vi "CRYGraph Digital Window.vi"() -> ()   [LabVIEW 2013]
uses:
  Control/CRYFlag Cluster.ctl
  <vilib>/Utility/miscctls.llb/LVRowAndColumnTypeDef.ctl
  <vilib>/Utility/miscctls.llb/LVRectTypeDef.ctl
  SubVI/CRYData View Global.vi
  SubVI/CRYMain Sub Window Global.vi
  CRYCurveLibrary/Global/CRYCurve Library Global.vi
panel:
  out "LegendVScrollShow":bool=TRUE
  in  "LoadFinish":bool
  in  "ScaleFitY":bool
  in  "ScaleFitX":bool
  in  "ToolbarUpdate":bool
  in  "PaletteShow":bool
  out "PropertyTab":string
  in  "OpenProperty":bool
  out "Event Name":string
  out "Test":string
  in  "Cursor":string[][](table)
  out "Cursor Ref":refnum<vi>
  out "Queue Name":string
  in  "StateOut":bool
  in  "CursorShow":bool
  out "Graph Ref":refnum<vi>
  out "Digital Graph":digitalwaveform[](graph)
  in  "LegendShow":bool
  out "Legend Ref":refnum<vi>
  out "Title Name":string
  out "OldRow":i32
  out "TotalPlot":u32
  out "Graph Number":i32
  in  "stop":bool
  in  "ColorBox":u32(colorbox)
  in  "Legend":i32(listbox)
  in  "GraphType":string
types:
  T1 = typedef "CRYFlag Cluster.ctl" = cluster{"LegendShow":bool, "CellClick":bool, "Total Number":bool, "ScaleFitX":bool, "ScaleFitY":bool, "MapModeX":u8, "MapModeY":u8, "CursorShow":bool, "MagnitudeShow":bool, "PreviewShow":bool, "CursorEnabled":bool, "IntensityShow":bool, "PaletteShow":bool, "PhaseShow":bool, "XYShow":bool, "FrequencyShow":bool, "LegendVScrollShow":bool, "FrequencyVScrollShow":bool}
  T2 = cluster{"DisplayTitle":string, "DataViewTitle":string, "DataType":string, "XAxisLabel":string, "YAxisLabel":string, "GraphData":variant}
  T3 = typedef "CRYGraph Event.ctl" = cluster{"EvenName":string, "TitleName":string, "GraphName":string, "GraphType":string, "Data":variant, "Queue Name":string, "DataView Number":i32}
  T4 = enum16{"Curves", "Values", "Results", "WFM", "Others"}
  T5 = typedef "LVRowAndColumnTypeDef.ctl" = cluster{"Row":i32, "Column":i32}
  T6 = typedef "LVRectTypeDef.ctl" = cluster{"Left":i16, "Top":i16, "Right":i16, "Bottom":i16}
  T7 = typedef "LVPoint32TypeDef.ctl" = cluster{"Horizontal":i32, "Vertical":i32}
  T8 = typedef "LVBoundsTypeDef.ctl" = cluster{"Width":u32, "Height":u32}
  T9 = typedef "LVPositionTypeDef.ctl" = cluster{"Left":i32, "Top":i32}
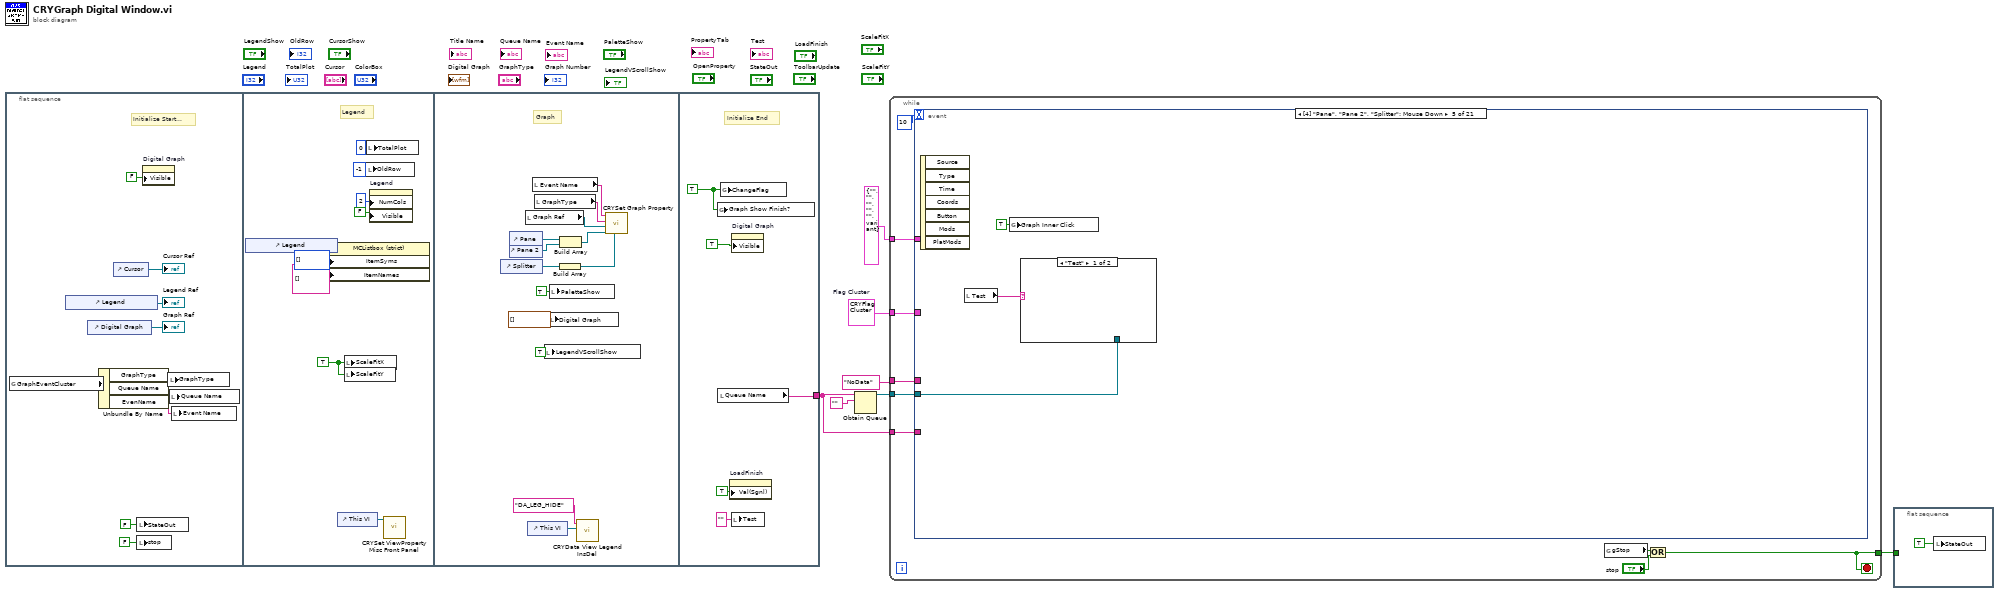
[diagram p0: block diagram]
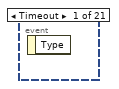
[diagram p2: hidden frame]
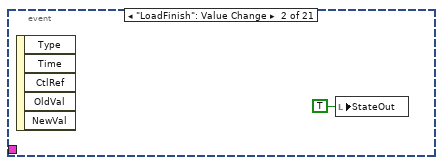
[diagram p3: hidden frame]
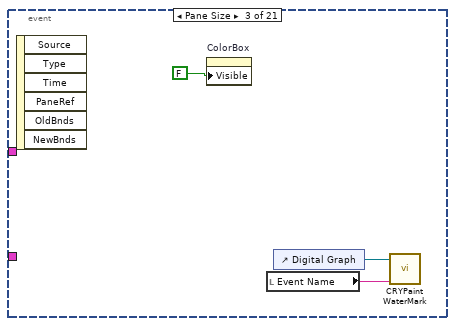
[diagram p4: hidden frame]
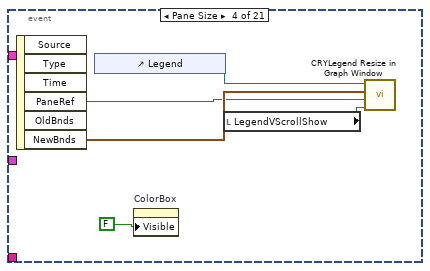
[diagram p5: hidden frame]
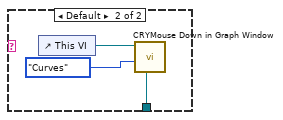
[diagram p6: hidden frame]
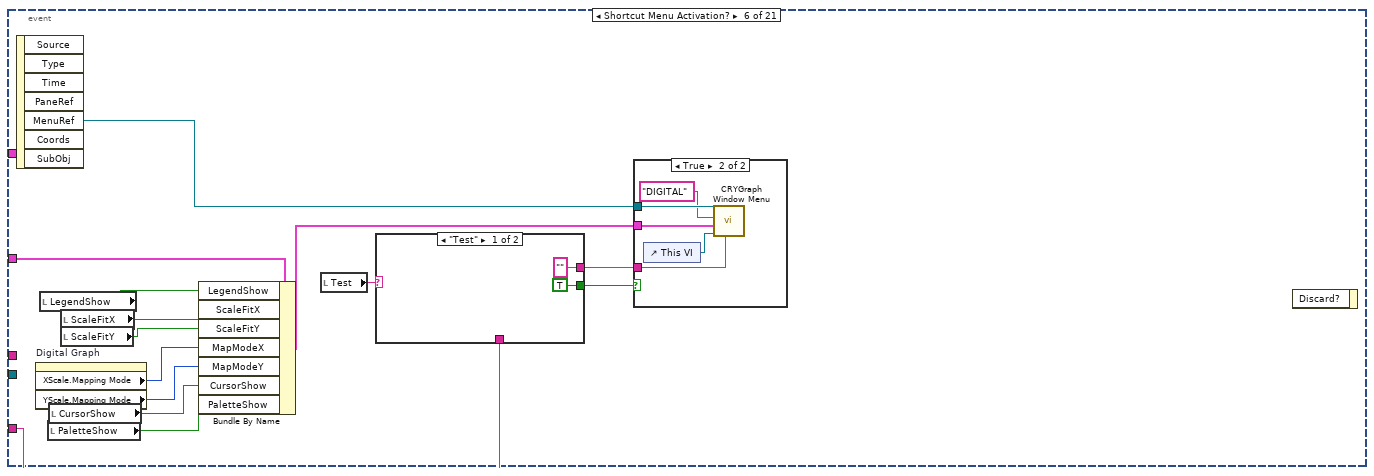
[diagram p7: hidden frame]
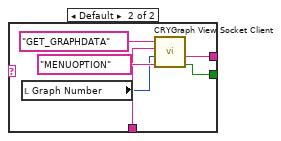
[diagram p8: hidden frame]
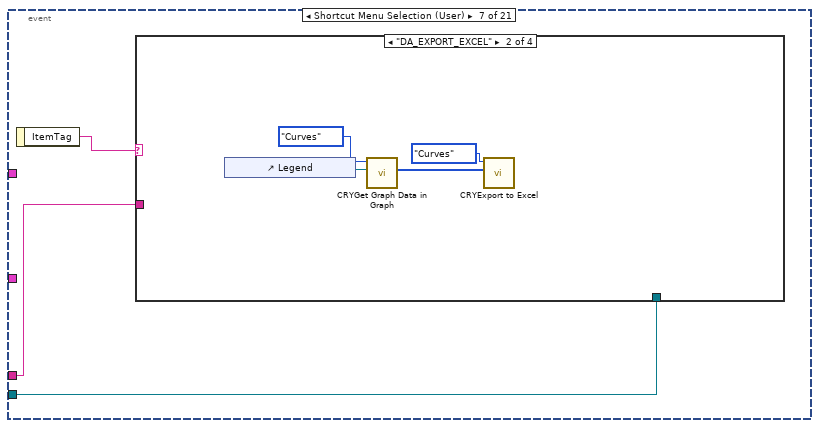
[diagram p10: hidden frame]
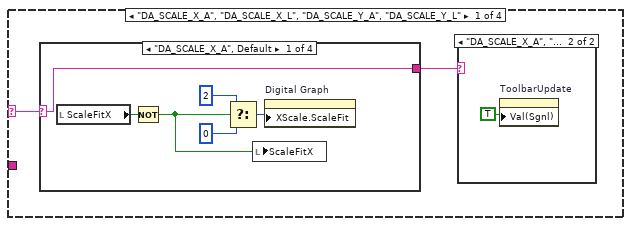
[diagram p11: hidden frame]
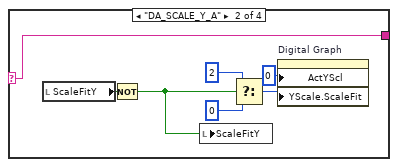
[diagram p13: hidden frame]
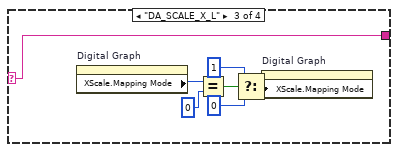
[diagram p14: hidden frame]
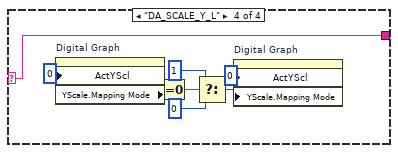
[diagram p15: hidden frame]
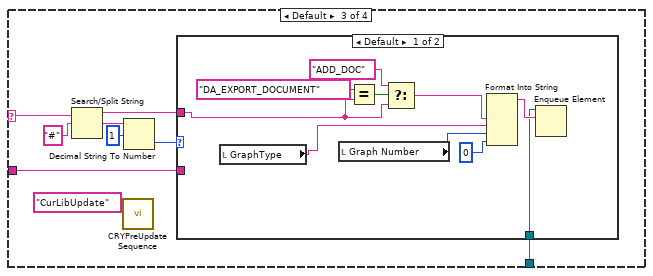
[diagram p16: hidden frame]
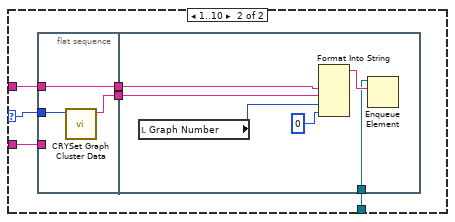
[diagram p17: hidden frame]
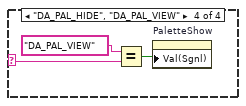
[diagram p18: hidden frame]
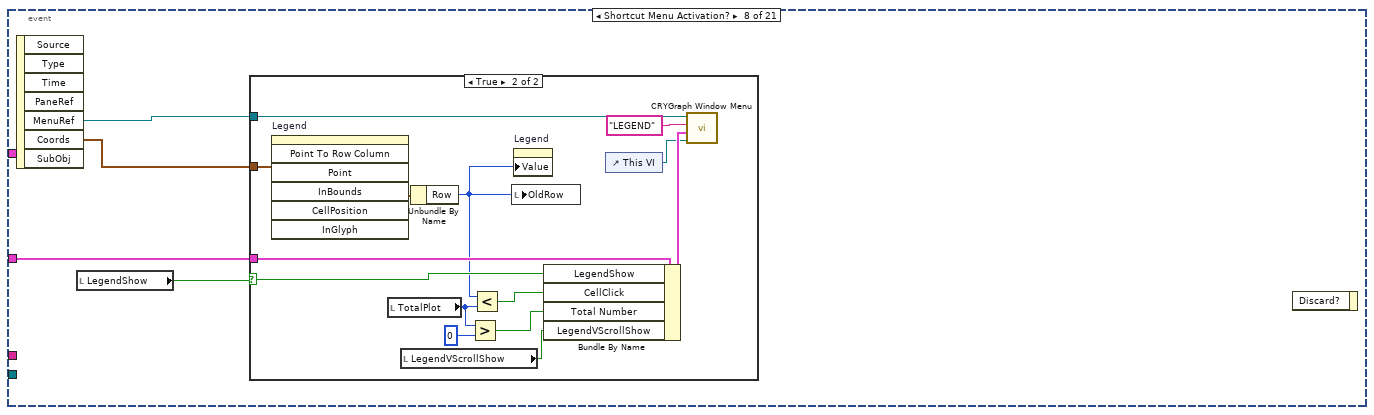
[diagram p19: hidden frame]
diagram:
  w4 = T1 {"LegendShow"=FALSE, "CellClick"=FALSE, "Total Number"=FALSE, "ScaleFitX"=FALSE, "ScaleFitY"=FALSE, "MapModeX"=0, "MapModeY"=0, "CursorShow"=FALSE, "MagnitudeShow"=FALSE, "PreviewShow"=FALSE, "CursorEnabled"=FALSE, "IntensityShow"=FALSE, "PaletteShow"=FALSE, "PhaseShow"=FALSE, "XYShow"=FALSE, "FrequencyShow"=FALSE, "LegendVScrollShow"=FALSE, "FrequencyVScrollShow"=FALSE}  # Flag Cluster
  n1 = flat-sequence {
    tunnel: [w41] -> w2
    frame #0 {
      # "Initialize Start..."
      n2 = global read "CRYData View Global.vi" "GraphEventCluster"() -> (w10:T3)
      n3 = control-ref of="Legend"() -> (→"Legend Ref":refnum<vi>)
      n4 = control-ref of="Digital Graph"() -> (→"Graph Ref":refnum<vi>)
      n5 = Unbundle By Name(w10) -> ("GraphType"=w9:string, "Queue Name"=w11:string, "EvenName"=w8:string)
      n6 = control-ref of="Cursor"() -> (→"Cursor Ref":refnum<vi>)
      n7 = local write "StateOut"(FALSE ("StateOut")) -> ()
      n8 = local write "stop"(FALSE ("stop")) -> ()
      n9 = property on="Digital Graph" class="DigitalGraph (strict)"("Visible"=FALSE) -> ()  [unwired: 2 in, 2 out]
      n10 = local write "GraphType"(w9) -> ()
      n11 = local write "Queue Name"(w11) -> ()
      n12 = local write "Event Name"(w8) -> ()
    }
    frame #1 {
      w18 = TRUE ("ScaleFitX")
      # "Legend"
      n13 = control-ref of="Legend"() -> (w20:refnum<vi>)
      n14 = property on="Property Node" class="MCListbox (strict)"(reference=w20, "ItemSyms"=i32[] [] ("Item Symbols"), "ItemNames"=string[][] [] ("Item Names")) -> ()  [unwired: 1 in, 2 out]
      n15 = control-ref of="This VI"() -> (w19:refnum<vi>)
      n16 = local write "ScaleFitX"(w18) -> ()
      n17 = local write "ScaleFitY"(w18) -> ()
      n18 = local write "OldRow"(-1 ("OldRow 2")) -> ()
      n19 = local write "TotalPlot"(u32 0 ("TotalPlot")) -> ()
      n20 = property on="Legend" class="MCListbox (strict)"("NumCols"=u32 2 ("Number of Columns"), "Visible"=FALSE) -> ()  [unwired: 2 in, 2 out]
      n21 = call "CRYSet ViewProperty Misc Front Panel.vi"("Vi Ref"=w19) -> ()  [unwired: 11 in]
    }
    frame #2 {
      # "Graph"
      n22 = control-ref of="Splitter"() -> (w33:refnum<vi>)
      n23 = control-ref of="Pane"() -> (w31:refnum<vi>)
      n24 = control-ref of="Pane 2"() -> (w32:refnum<vi>)
      n25 = local read "Graph Ref"() -> (w36:refnum<vi>)
      n26 = control-ref of="This VI"() -> (w37:refnum<vi>)
      n27 = local read "Event Name"() -> (w29:string)
      n28 = local read "GraphType"() -> (w30:string)
      n29 = local write "LegendVScrollShow"(TRUE ("LegendVScrollShow")) -> ()
      n30 = local write "Digital Graph"(digitalwaveform[] [] ("Digital Graph")) -> ()
      n31 = local write "PaletteShow"(TRUE ("PaletteShow")) -> ()
      n32 = Build Array(w33) -> (w35:refnum<vi>[])
      n33 = Build Array(w31, w32) -> (w34:refnum<vi>[])
      n34 = call "CRYData View Legend InsDel.vi"("Graph VI Ref"=w37, "sAction"="DA_LEG_HIDE" ("Action Type")) -> ()  [unwired: 2 in, 8 out]
      n35 = call "CRYSet Graph Property.vi"("Splitters"=w35, "Panes"=w34, "Graph Ref"=w36, "Graph Type"=w30, "Event Name"=w29) -> ()  [unwired: 7 in]
    }
    frame #3 {
      w44 = TRUE ("ChangeFlag")
      # "Initialize End"
      n36 = global write "CRYData View Global.vi" "Graph Show Finish?"(w44) -> ()
      n37 = local read "Queue Name"() -> (w41:string)
      n38 = global write "CRYData View Global.vi" "ChangeFlag"(w44) -> ()
      n39 = property on="LoadFinish" class="Bool (strict)"("Val(Sgnl)"=TRUE ("Value (Signaling)")) -> ()  [unwired: 2 in, 2 out]
      n40 = local write "Test"("" ("Test")) -> ()
      n41 = property on="Digital Graph" class="DigitalGraph (strict)"("Visible"=TRUE) -> ()  [unwired: 2 in, 2 out]
    }
  }
  n42 = Obtain Queue(name (unnamed)=w2, element data type="") -> (queue out=w7:refnum<queue>)  [unwired: 3 in, 2 out]
  n43 = while {
    tunnel: w7 -> [w53]
    tunnel: T2 {"DisplayTitle"="", "DataViewTitle"="", "DataType"="", "XAxisLabel"="", "YAxisLabel"="", "GraphData"=variant} ("Graph Cluster") -> [w51]
    tunnel: w4 -> [w50]
    tunnel: "NoData" ("input 2") -> [w47]
    tunnel: w2 -> [w46]
    tunnel: [w45] -> w1
    stop <- w45 stop-if-true
    n44 = event shown="[4] \"Pane\", \"Pane 2\", \"Splitter\": Mouse Down" {
      selector: _ -> [_ _ _ _ _ _ _ _ _ _ _ _ _ _ _ _ _ _ _ _ _]
      dyn-events: _ -> [_ _ _ _ _ _ _ _ _ _ _ _ _ _ _ _ _ _ _ _ _]
      timeout: 10 -> [_ _ _ _ _ _ _ _ _ _ _ _ _ _ _ _ _ _ _ _ _]
      tunnel: w51 -> [_ _ _ _ _ _ _ _ _ _ _ _ _ _ _ _ _ _ _ _ _]
      tunnel: w53 -> [_ _ _ _ w65 _ w98 _ w192 _ _ _ _ _ _ _ _ w328 _ _ _]
      tunnel: w50 -> [_ _ _ _ _ w82 _ w172 _ _ _ _ _ _ _ _ _ _ _ _ _]
      tunnel: w47 -> [_ _ _ _ _ _ w96 _ w189 _ _ _ _ _ _ _ _ _ _ _ _]
      tunnel: w46 -> [_ _ _ _ _ w76 _ _ _ _ _ _ _ _ w300 _ _ _ _ _ _]
      event Timeout {
        n45 = event-data() -> ()  [unwired: 2 out]
      }
      event "LoadFinish": Value Change {
        n46 = event-data() -> ()  [unwired: 6 out]
        n47 = local write "StateOut"(TRUE ("StateOut")) -> ()
      }
      event Pane Size {
        n48 = event-data() -> ()  [unwired: 7 out]
        n49 = property on="ColorBox" class="ColBox"("Visible"=FALSE) -> ()  [unwired: 2 in, 2 out]
        n50 = local read "Event Name"() -> (w55:string)
        n51 = control-ref of="Digital Graph"() -> (w56:refnum<vi>)
        n52 = call "CRYPaint WaterMark.vi"("Type"=w55, "Graph Ref"=w56) -> ()  [unwired: 10 in]
      }
      event Pane Size {
        n53 = event-data() -> ("PaneRef"=w59:refnum<vi>, "NewBnds"=w60:T6)  [unwired: 5 out]
        n54 = control-ref of="Legend"() -> (w61:refnum<vi>)
        n55 = property on="ColorBox" class="ColBox"("Visible"=FALSE) -> ()  [unwired: 2 in, 2 out]
        n56 = local read "LegendVScrollShow"() -> (w58:bool)
        n57 = call "CRYLegend Resize in Graph Window.vi"("VScrollShow"=w58, "Pane Ref"=w59, "input cluster"=w60, "Legend"=w61) -> ()  [unwired: 8 out]
      }
      event Mouse Down {
        n58 = event-data() -> ()  [unwired: 8 out]
        n59 = local read "Test"() -> (w64:string)
        n60 = global write "CRYCurve Library Global.vi" "Graph Inner Click"(TRUE ("Graph Inner Click")) -> ()
        n61 = case shown="\"Test\"" w64 {
          tunnel: w65 -> [_ w67]
          frame "Test" {
          }
          frame Default {
            n62 = control-ref of="This VI"() -> (w66:refnum<vi>)
            n63 = call "CRYMouse Down in Graph Window.vi"("Queue"=w67, "Selected Type"=enum16{"Curves", "Values", "Results", "WFM"}."Curves" ("Type"), "pGraph VI In"=w66) -> ()  [unwired: 3 in, 6 out]
          }
        }
      }
      event Shortcut Menu Activation? {
        n64 = event-data() -> ("MenuRef"=w77:refnum<k9>)  [unwired: 7 out]
        n65 = property on="Digital Graph" class="DigitalGraph (strict)"() -> ("XScale.Mapping Mode"=w74:u8, "YScale.Mapping Mode"=w73:u8)  [unwired: 2 in, 2 out]
        n66 = local read "LegendShow"() -> (w81:bool)
        n67 = local read "PaletteShow"() -> (w71:bool)
        n68 = local read "CursorShow"() -> (w72:bool)
        n69 = local read "ScaleFitX"() -> (w70:bool)
        n70 = local read "ScaleFitY"() -> (w69:bool)
        n71 = Bundle By Name(cluster=w82, "LegendShow"=w81, "ScaleFitX"=w70, "ScaleFitY"=w69, "MapModeX"=w74, "MapModeY"=w73, "CursorShow"=w72, "PaletteShow"=w71) -> (w78:T1)
        n72 = local read "Test"() -> (w75:string)
        n73 = case shown="\"Test\"" w75 {
          tunnel: ["" ("sData Out") w88] -> w80
          tunnel: [TRUE ("bResult Out") w87] -> w79
          tunnel: w76 -> [_ w86]
          frame "Test" {
          }
          frame Default {
            n74 = local read "Graph Number"() -> (w85:i32)
            n75 = call "CRYGraph View Socket Client.vi"("sOption"="MENUOPTION", "nData"=w85, "sData"=w86, "sAction"="GET_GRAPHDATA") -> ("bResult Out"=w87:bool, "sData Out"=w88:string)  [unwired: 4 in, 2 out]
          }
        }
        n76 = case shown="True" w79 {
          tunnel: w77 -> [_ w95]
          tunnel: w78 -> [_ w93]
          tunnel: w80 -> [_ w92]
          frame False {
          }
          frame True {
            n77 = control-ref of="This VI"() -> (w91:refnum<vi>)
            n78 = call "CRYGraph Window Menu.vi"("MenuOption"=w92, "pGraph VI"=w91, "Flag Cluster"=w93, "Type"="DIGITAL", "Runtime Menu Ref In"=w95) -> ()  [unwired: 7 out]
          }
        }
        n79 = event-data() -> ()  [unwired: 1 in, 2 out]
      }
      event Shortcut Menu Selection (User) {
        n80 = event-data() -> ("ItemTag"=w97:string)  [unwired: 1 out]
        n81 = case shown="\"DA_EXPORT_EXCEL\"" w97 {
          selector: w97 -> [w100 _ w137 w169]
          tunnel: w98 -> [_ _ w136 _]
          tunnel: w96 -> [_ _ w135 _]
          frame "DA_SCALE_X_A", "DA_SCALE_X_L", "DA_SCALE_Y_A", "DA_SCALE_Y_L" {
            n82 = case shown="\"DA_SCALE_X_A\", Default" w100 {
              selector: w100 -> [w104 w111 w115 w124]
              tunnel: [w104 w111 w115 w124] -> w99
              frame "DA_SCALE_X_A", Default {
                n83 = local read "ScaleFitX"() -> (w103:bool)
                n84 = Not(x=w103) -> (.not. x?=w102:bool)
                n85 = Select(t=u8 2, s=w102, f=u8 0) -> (s? t:f=w105:u8)
                n86 = local write "ScaleFitX"(w102) -> ()
                n87 = property on="Digital Graph" class="DigitalGraph (strict)"("XScale.ScaleFit"=w105) -> ()  [unwired: 2 in, 2 out]
              }
              frame "DA_SCALE_Y_A" {
                n88 = local read "ScaleFitY"() -> (w109:bool)
                n89 = Not(x=w109) -> (.not. x?=w108:bool)
                n90 = local write "ScaleFitY"(w108) -> ()
                n91 = Select(t=u8 2, s=w108, f=u8 0) -> (s? t:f=w112:u8)
                n92 = property on="Digital Graph" class="DigitalGraph (strict)"("ActYScl"=0 ("Active Y Scale"), "YScale.ScaleFit"=w112) -> ()  [unwired: 2 in, 2 out]
              }
              frame "DA_SCALE_X_L" {
                n93 = property on="Digital Graph" class="DigitalGraph (strict)"() -> ("XScale.Mapping Mode"=w117:u8)  [unwired: 2 in, 2 out]
                n94 = Equal?(x=w117, y=u8 0) -> (x = y?=w121:bool)
                n95 = Select(t=u8 1, s=w121, f=u8 0) -> (s? t:f=w116:u8)
                n96 = property on="Digital Graph" class="DigitalGraph (strict)"("XScale.Mapping Mode"=w116) -> ()  [unwired: 2 in, 2 out]
              }
              frame "DA_SCALE_Y_L" {
                n97 = property on="Digital Graph" class="DigitalGraph (strict)"("ActYScl"=0 ("Active Y Scale")) -> ("YScale.Mapping Mode"=w126:u8)  [unwired: 2 in, 2 out]
                n98 = Equal To 0?(x=w126) -> (x = 0?=w129:bool)
                n99 = Select(t=u8 1, s=w129, f=u8 0) -> (s? t:f=w125:u8)
                n100 = property on="Digital Graph" class="DigitalGraph (strict)"("ActYScl"=0 ("Active Y Scale"), "YScale.Mapping Mode"=w125) -> ()  [unwired: 2 in, 2 out]
              }
            }
            n101 = case shown="\"DA_SCALE_X_A\", \"DA_SCALE_Y_A\"" w99 {
              frame Default {
              }
              frame "DA_SCALE_X_A", "DA_SCALE_Y_A" {
                n102 = property on="ToolbarUpdate" class="Bool (strict)"("Val(Sgnl)"=TRUE ("Value (Signaling)")) -> ()  [unwired: 2 in, 2 out]
              }
            }
          }
          frame "DA_EXPORT_EXCEL" {
            n103 = control-ref of="Legend"() -> (w131:refnum<vi>)
            n104 = call "CRYGet Graph Data in Graph.vi"("Legend Refnum"=w131, "Type In"=enum16{"Curves", "Values", "Results", "WFM"}."Curves" ("Type")) -> ("Rows"=w130:i32[])  [unwired: 2 in, 7 out]
            n105 = call "CRYExport to Excel.vi"("Rows"=w130, "Type"=T4."Curves") -> ()  [unwired: 2 in, 8 out]
          }
          frame Default {
            n106 = Search/Split String(string=w137, search string/char (-)="#") -> (substring before match=w140:string, match + rest of string=w139:string)  [unwired: 2 out]
            n107 = call "CRYPreUpdate Sequence.vi"("EventName"="CurLibUpdate") -> ()  [unwired: 15 in]
            n108 = Decimal String To Number(string=w139, offset=1) -> (number=w141:i32)  [unwired: 2 out]
            n109 = case shown="Default" w141 {
              selector: w141 -> [_ w158]
              tunnel: w140 -> [w145 w156]
              tunnel: w136 -> [w150 w155]
              tunnel: w135 -> [_ w153]
              frame Default {
                n110 = local read "GraphType"() -> (w143:string)
                n111 = local read "Graph Number"() -> (w149:i32)
                n112 = Equal?(x="DA_EXPORT_DOCUMENT" ("y"), y=w145) -> (x = y?=w148:bool)
                n113 = Select(t="ADD_DOC", s=w148, f=w145) -> (s? t:f=w144:string)
                n114 = Format Into String(w144, w143, w149, 0 ("input 3")) -> (resulting string=w151:string)  [unwired: 3 in, 1 out]
                n115 = Enqueue Element(queue=w150, element=w151) -> ()  [unwired: 1 in, 4 out]
              }
              frame 1..10 {
                n116 = flat-sequence {
                  tunnel: w158 -> [w161]
                  tunnel: [w160] -> w157
                  tunnel: w156 -> [w160]
                  tunnel: [w159] -> w154
                  tunnel: w153 -> [_]
                  tunnel: w157 -> [w165]
                  tunnel: w155 -> [w164]
                  tunnel: w154 -> [w163]
                  frame #0 {
                    n117 = call "CRYSet Graph Cluster Data.vi"("Graph Number"=w161) -> ("DataType"=w159:string)  [unwired: 2 in, 8 out]
                  }
                  frame #1 {
                    n118 = local read "Graph Number"() -> (w162:i32)
                    n119 = Format Into String(w165, w163, w162, 0 ("input 3")) -> (resulting string=w167:string)  [unwired: 3 in, 1 out]
                    n120 = Enqueue Element(queue=w164, element=w167) -> ()  [unwired: 1 in, 4 out]
                  }
                }
              }
            }
          }
          frame "DA_PAL_HIDE", "DA_PAL_VIEW" {
            n121 = Equal?(x="DA_PAL_VIEW" ("y"), y=w169) -> (x = y?=w168:bool)
            n122 = property on="PaletteShow" class="Bool (strict)"("Val(Sgnl)"=w168) -> ()  [unwired: 2 in, 2 out]
          }
        }
      }
      event Shortcut Menu Activation? {
        n123 = event-data() -> ("MenuRef"=w173:refnum<k9>, "Coords"=w174:T7)  [unwired: 6 out]
        n124 = local read "LegendShow"() -> (w171:bool)
        n125 = case shown="True" w171 {
          selector: w171 -> [_ w177]
          tunnel: w174 -> [_ w187]
          tunnel: w173 -> [_ w185]
          tunnel: w172 -> [_ w183]
          frame False {
          }
          frame True {
            n126 = invoke on="Legend" class="MCListbox (strict)" method="Point To Row Column"("Point"=w187) -> ("CellPosition"=w188:T5)  [unwired: 6 in, 6 out]
            n127 = local read "TotalPlot"() -> (w179:u32)
            n128 = local read "LegendVScrollShow"() -> (w175:bool)
            n129 = Unbundle By Name(w188) -> ("Row"=w176:i32)
            n130 = Greater?(x=w179, y=u32 0) -> (0:w181:bool)
            n131 = Less?(x=w176, y=w179) -> (x < y?=w182:bool)
            n132 = local write "OldRow"(w176) -> ()
            n133 = property on="Legend" class="MCListbox (strict)"("Value"=w176) -> ()  [unwired: 2 in, 2 out]
            n134 = Bundle By Name(cluster=w183, "LegendShow"=w177, "CellClick"=w182, "Total Number"=w181, "LegendVScrollShow"=w175) -> (w180:T1)
            n135 = control-ref of="This VI"() -> (w178:refnum<vi>)
            n136 = call "CRYGraph Window Menu.vi"("pGraph VI"=w178, "Flag Cluster"=w180, "Type"="LEGEND", "Runtime Menu Ref In"=w185) -> ()  [unwired: 1 in, 7 out]
          }
        }
        n137 = event-data() -> ()  [unwired: 1 in, 2 out]
      }
      event Shortcut Menu Selection (User) {
        n138 = event-data() -> ("ItemTag"=w193:string)  [unwired: 8 out]
        n139 = local read "Graph Number"() -> (w190:i32)
        n140 = case shown="\"DA_LEG_REMOVEALL\"" w193 {
          selector: w193 -> [_ _ _ _ _ w244]
          tunnel: w192 -> [_ w198 _ _ _ _]
          tunnel: w190 -> [_ w197 _ _ _ _]
          tunnel: w189 -> [_ w194 _ _ _ _]
          frame Default {
          }
          frame "DA_LEG_HIDE_1" {
            n141 = Format Into String("DA_LEG_HIDE" ("input 2"), w194, w197, 0 ("input 3")) -> (resulting string=w199:string)  [unwired: 3 in, 1 out]
            n142 = Enqueue Element(queue=w198, element=w199) -> ()  [unwired: 1 in, 4 out]
          }
          frame "DA_LEG_REMOVE" {
            n143 = flat-sequence {
              tunnel: [w203] -> w200
              tunnel: w200 -> [w212]
              frame #0 {
                n144 = control-ref of="Legend"() -> (w206:refnum<vi>)
                n145 = local read "TotalPlot"() -> (w210:u32)
                n146 = local read "GraphType"() -> (w205:string)
                n147 = local read "OldRow"() -> (w203:i32)
                n148 = Decrement(x=w210) -> (x-1=w211:u32)
                n149 = local write "TotalPlot"(w211) -> ()
                n150 = Build Array(w203) -> (w202:i32[])
                n151 = call "CRYData View Legend Manipulate.vi"("sAction"="GetGlobalNumbyLegNum", "nData"=w202, "sData"=w205, "Legend Ref"=w206) -> ("nData Out"=w204:i32[])  [unwired: 6 in, 1 out]
                n152 = control-ref of="This VI"() -> (w208:refnum<vi>)
                n153 = call "CRYSymbol Conversion.vi"("pGraph VI"=w208, "CurLib Tab Type"=enum16{"Curves", "Values", "Results", "WFM"}."Curves", "nDatas"=w204, "sActin"="LEGEND_REMOVE") -> ()  [unwired: 8 in]
              }
              frame #1 {
                n154 = control-ref of="Legend"() -> (w213:refnum<vi>)
                n155 = call "CRYData View Legend Item Delete.vi"("RowNumber"=w212, "Legend MultiListbox In"=w213) -> ()  [unwired: 10 out]
              }
              frame #2 {
                n156 = local read "TotalPlot"() -> (w214:u32)
                n157 = case shown="1, Default" w214 {
                  selector: w214 -> [_ w219]
                  frame 0 {
                    n158 = local write "GraphType"("EMPTY" ("Data Type")) -> ()
                  }
                  frame 1, Default {
                    n159 = for {
                      N: w219 -> [_]
                      i -> [w224]
                      n160 = property on="Legend" class="MCListbox (strict)"() -> ("ItemSyms"=w225:i32[])  [unwired: 2 in, 2 out]
                      n161 = Bundle By Name(cluster=T5 {"Row"=0, "Column"=0} ("Active Cell:Active Cell"), "Row"=w224, "Column"=1) -> (w226:T5)
                      n162 = Index Array(array=w225, index=w224) -> (element=w222:i32)
                      n163 = property on="Legend" class="MCListbox (strict)"("ActiveCell"=w226) -> ("CellBG"=w221:u32)  [unwired: 2 in, 2 out]
                      n164 = Equal?(x=w222, y=38) -> (x = y?=w220:bool)
                      n165 = property on="Digital Graph" class="DigitalGraph (strict)"("Active Plot"=w224, "Plot.Plot Color"=w221, "Plot.Fill/Pt. Color"=w221, "Plot.Visible?"=w220) -> ()  [unwired: 2 in, 2 out]
                    }
                  }
                }
                n166 = local read "Digital Graph"() -> (w215:digitalwaveform[])
                n167 = local read "OldRow"() -> (w217:i32)
                n168 = Delete From Array(array=w215, index=w217) -> (array with subset deleted=w216:digitalwaveform[])  [unwired: 1 in, 1 out]
                n169 = local write "Digital Graph"(w216) -> ()
              }
            }
          }
          frame "DA_LEG_REMOVEALL" {
            n170 = flat-sequence {
              frame #0 {
                n171 = control-ref of="This VI"() -> (w233:refnum<vi>)
                n172 = Build Array(-1 ("nData")) -> (w234:i32[])
                n173 = call "CRYSymbol Conversion.vi"("pGraph VI"=w233, "CurLib Tab Type"=enum16{"Curves", "Values", "Results", "WFM"}."Curves", "nDatas"=w234, "sActin"="LEGEND_REMOVE") -> ()  [unwired: 8 in]
              }
              frame #1 {
                n174 = control-ref of="Legend"() -> (w237:refnum<vi>)
                n175 = call "CRYData View Legend Item Delete.vi"("RowNumber"=-1, "Legend MultiListbox In"=w237) -> ()  [unwired: 10 out]
              }
            }
            n176 = local write "TotalPlot"(u32 0 ("TotalPlot")) -> ()
            n177 = local write "Digital Graph"(digitalwaveform[] [] ("Digital Graph")) -> ()
          }
          frame "DA_LEG_INVERT" {
            n178 = local read "TotalPlot"() -> (w239:u32)
            n179 = for {
              N: w239 -> [_]
              tunnel: [38] -> w238 mode=indexing
              i -> [w242]
              n180 = property on="Digital Graph" class="DigitalGraph (strict)"("Active Plot"=w242, "Plot.Visible?"=TRUE ("Plot.Visible")) -> ()  [unwired: 2 in, 2 out]
            }
            n181 = property on="Legend" class="MCListbox (strict)"("ItemSyms"=w238) -> ()  [unwired: 2 in, 2 out]
          }
          frame "DA_LEG_VSCROLL_HIDE", "DA_LEG_VSCROLL_VIEW" {
            n182 = Equal?(x="DA_LEG_VSCROLL_VIEW" ("y"), y=w244) -> (x = y?=w243:bool)
            n183 = property on="LegendVScrollShow" class="Bool (strict)"("Val(Sgnl)"=w243) -> ()  [unwired: 2 in, 2 out]
          }
        }
        n184 = call "CRYPreUpdate Sequence.vi"("EventName"="CurLibUpdate") -> ()  [unwired: 15 in]
      }
      event "PaletteShow": Value Change {
        n185 = event-data() -> ("NewVal"=w246:bool)  [unwired: 6 out]
        n186 = property on="Digital Graph" class="DigitalGraph (strict)"("Palette Visible"=w246) -> ()  [unwired: 2 in, 2 out]
      }
      event "Legend": Mouse Down {
        n187 = event-data() -> ("CtlRef"=w248:refnum<vi>, "Coords"=w253:T7, "Button"=w252:u16)  [unwired: 6 out]
        n188 = local read "TotalPlot"() -> (w247:u32)
        n189 = call "CRYData View Legend Plot OnOff.vi"("TotalPlot"=w247, "Button Info"=w252, "Mouse Point"=w253, "MCListbox Ref In"=w248) -> ("Active Row"=w249:i32, "Visible?"=w250:bool, "Click State"=w251:bool)  [unwired: 5 out]
        n190 = case shown="True" w251 {
          tunnel: w250 -> [_ w256]
          tunnel: w249 -> [_ w257]
          frame False {
          }
          frame True {
            n191 = flat-sequence {
              tunnel: w257 -> [w259]
              tunnel: w256 -> [w258]
              tunnel: [w258] -> w254
              tunnel: [w260] -> w255
              tunnel: w254 -> [w260]
              frame #0 {
                n192 = property on="Digital Graph" class="DigitalGraph (strict)"("Active Plot"=w259) -> ()  [unwired: 2 in, 2 out]
              }
              frame #1 {
                n193 = property on="Digital Graph" class="DigitalGraph (strict)"("Plot.Visible?"=w260) -> ()  [unwired: 2 in, 2 out]
              }
            }
            n194 = disable-structure shown="Disabled" {
              disable-tunnel: w255 -> [w261 _]
              frame Disabled {
                n195 = case shown="True" w261 {
                  frame False {
                  }
                  frame True {
                    n196 = property on="Digital Graph" class="DigitalGraph (strict)"("Active Plot"=u32 0) -> ()  [unwired: 2 in, 2 out]
                  }
                }
              }
              frame Enabled {
              }
            }
          }
        }
      }
      event "Legend": Mouse Move {
        n197 = event-data() -> ("Coords"=w263:T7)  [unwired: 5 out]
        n198 = control-ref of="Legend"() -> (w265:refnum<vi>)
        n199 = local read "TotalPlot"() -> (w264:u32)
        n200 = call "CRYData View Legend Mouse Move.vi"("TotalPlot"=w264, "Mouse Point"=w263, "MCListbox Ref In"=w265) -> ("CellSize"=w267:T8, "Position"=w268:T9, "Selected Row"=w269:i32, "Move State"=w270:bool, "CellBG"=w266:u32)  [unwired: 1 in, 3 out]
        n201 = case shown="True" w270 {
          tunnel: w266 -> [_ w275]
          tunnel: w267 -> [_ w274]
          tunnel: w268 -> [_ w273]
          tunnel: w269 -> [_ w272]
          frame False {
            n202 = property on="ColorBox" class="ColBox"("Visible"=FALSE) -> ()  [unwired: 2 in, 2 out]
          }
          frame True {
            n203 = local write "OldRow"(w272) -> ()
            n204 = property on="ColorBox" class="ColBox"("Position"=w273, "Color Area Size"=w274, "Value"=w275) -> ()  [unwired: 2 in, 2 out]
            n205 = property on="ColorBox" class="ColBox"("Visible"=TRUE) -> ()  [unwired: 2 in, 2 out]
          }
        }
      }
      event "Legend": Double Click {
        n206 = event-data() -> ("CtlRef"=w277:refnum<vi>, "Coords"=w278:T7)  [unwired: 8 out]
        n207 = disable-structure shown="Disabled" {
          disable-tunnel: w278 -> [w284 _]
          disable-tunnel: w277 -> [w283 _]
          frame Disabled {
            n208 = call "CRYGet MultiListBox Click State.vi"("Coords"=w284, "MultiList Box Ref In"=w283) -> ("State"=w282:bool)  [unwired: 6 in, 3 out]
            n209 = call "CRYClick Name in Legend.vi"("Mouse Point"=w284, "MCListbox Ref In"=w283) -> ("Active Row"=w279:i32, "Click State?"=w281:bool)  [unwired: 8 in]
            n210 = And(x=w282, y=w281) -> (x .and. y?=w280:bool)
            n211 = case shown="True" w280 {
              tunnel: w283 -> [_ w287]
              tunnel: w279 -> [_ w286]
              frame False {
              }
              frame True {
                n212 = call "CRYOpen Step by Legend.vi"("Active Row"=w286, "MCListbox Ref In"=w287, "Type"=enum16{"Curves", "Values", "Results", "WFM"}."Curves" ("Type In")) -> ()  [unwired: 9 in]
              }
            }
          }
          frame Enabled {
          }
        }
      }
      event "LegendVScrollShow": Value Change {
        w299 = T6 {"Left"=0, "Top"=0, "Right"=0, "Bottom"=0}  # input cluster
        n213 = event-data() -> ("NewVal"=w290:bool)  [unwired: 6 out]
        n214 = property on="Legend" class="MCListbox (strict)"("VScrollVis"=w290) -> ()  [unwired: 2 in, 2 out]
        n215 = control-ref of="Pane 2"() -> (w291:refnum<vi>)
        n216 = property class="Pane"(reference=w291) -> ("Left"=w298:i32, "Top"=w295:i32, "Width"=w297:u32, "Height"=w294:u32)  [unwired: 1 in, 2 out]
        n217 = Add(x=w298, y=w297) -> (x+y=w296:u32)
        n218 = Add(x=w295, y=w294) -> (x+y=w293:u32)
        n219 = Bundle By Name(cluster=w299, "Left"=w298, "Top"=w295, "Right"=w296, "Bottom"=w293) -> (w292:T6)
        n220 = control-ref of="Legend"() -> (w289:refnum<vi>)
        n221 = local read "LegendVScrollShow"() -> (w288:bool)
        n222 = call "CRYLegend Resize in Graph Window.vi"("VScrollShow"=w288, "Pane Ref"=w291, "input cluster"=w292, "Legend"=w289) -> ()  [unwired: 8 out]
      }
      event "ColorBox": Value Change {
        # "Graph Color Changing"
        n223 = event-data() -> ("NewVal"=w302:u32)  [unwired: 6 out]
        n224 = local read "OldRow"() -> (w303:i32)
        n225 = flat-sequence {
          tunnel: [w311] -> w304
          tunnel: w302 -> [w311]
          tunnel: w303 -> [w310]
          tunnel: w304 -> [w313]
          frame #0 {
            n226 = property on="Digital Graph" class="DigitalGraph (strict)"("Active Plot"=w310) -> ()  [unwired: 2 in, 2 out]
            n227 = property on="Legend" class="MCListbox (strict)"("CellBG"=w311) -> ()  [unwired: 2 in, 2 out]
          }
          frame #1 {
            n228 = property on="Digital Graph" class="DigitalGraph (strict)"("Plot.Plot Color"=w313) -> ()  [unwired: 2 in, 2 out]
            n229 = property on="ColorBox" class="ColBox"("Visible"=FALSE) -> ()  [unwired: 2 in, 2 out]
          }
        }
        n230 = case shown="\"ViewReport\"" w300 {
          tunnel: w303 -> [_ w308]
          tunnel: w302 -> [_ w307]
          frame "ViewReport" {
          }
          frame Default {
            n231 = control-ref of="Legend"() -> (w306:refnum<vi>)
            n232 = call "CRYSet Plot Settings.vi"("sAction"="Color", "Color"=w307, "Row"=w308, "Legend Refnum"=w306, "Type"=enum16{"Curves", "Values", "Results", "WFM"}."Curves") -> ()  [unwired: 2 in, 5 out]
          }
        }
        n233 = call "CRYPreUpdate Sequence.vi"("EventName"="CurLibUpdate") -> ()  [unwired: 15 in]
      }
      event "ColorBox": Mouse Down {
        n234 = event-data() -> ()  [unwired: 9 out]
        n235 = local read "OldRow"() -> (w317:i32)
        n236 = Bundle By Name(cluster=T5 {"Row"=0, "Column"=0} ("Active Cell:Active Cell"), "Row"=w317, "Column"=1) -> (w314:T5)
        n237 = property on="Legend" class="MCListbox (strict)"("ActiveCell"=w314) -> ()  [unwired: 2 in, 2 out]
      }
      event "Digital Graph": Drag Enter {
        n238 = event-data() -> ("Available Data Names"=w319:string[])  [unwired: 1 out]
        n239 = disable-structure shown="Disabled" {
          disable-tunnel: w319 -> [w321 _]
          disable-tunnel: [w320 TRUE] -> w318
          frame Disabled {
            n240 = Search 1D Array(1D array=w321, element="CRY_GRAPH_DATA") -> (index of element=w323:i32)  [unwired: 1 out]
            n241 = Not Equal?(x=w323, y=-1) -> (x != y?=w320:bool)
          }
          frame Enabled {
          }
        }
        n242 = event-data("Accepted?"=w318) -> ()  [unwired: 1 in, 1 out]
      }
      event "Digital Graph": Drop {
        n243 = event-data() -> ()  [unwired: 2 out]
        n244 = local read "Event Name"() -> (w326:string)
        n245 = local read "TotalPlot"() -> (w331:u32)
        n246 = control-ref of="This VI"() -> (w327:refnum<vi>)
        n247 = call "CRYDrop Data in Same Graph.vi"("pGraph VI"=w327, "Queue"=w328, "Total Plot In"=w331, "sAction"=w326) -> ("Accepted?"=w329:bool, "Total Plot Out"=w330:u32)  [unwired: 3 in, 3 out]
        n248 = local write "TotalPlot"(w330) -> ()
        n249 = event-data("Accepted?"=w329) -> ()  [unwired: 1 in, 1 out]
      }
      event "Digital Graph": Scale Range Change {
        n250 = event-data() -> ("Kind"=w332:enum16{"X-Scale", "Y-Scale", "Z-Scale"})  [unwired: 5 out]
        n251 = case shown="\"Y-Scale\"" w332 {
          frame "X-Scale", Default {
            n252 = property on="Digital Graph" class="DigitalGraph (strict)"("XScale.ScaleFit"=u8 0 ("X Scale.Scale Fit")) -> ()  [unwired: 2 in, 2 out]
          }
          frame "Y-Scale" {
            n253 = property on="Digital Graph" class="DigitalGraph (strict)"("YScale.ScaleFit"=u8 0 ("Y Scale.Scale Fit")) -> ()  [unwired: 2 in, 2 out]
          }
        }
      }
      event "OpenProperty": Value Change {
        n254 = event-data() -> ()  [unwired: 7 out]
        n255 = flat-sequence {
          frame #0 {
            n256 = local read "PropertyTab"() -> (w335:string)
            n257 = control-ref of="This VI"() -> (w336:refnum<vi>)
            n258 = call "CRYGraph Property Window Main.vi"("TabName"=w335, "pGraph VI In"=w336) -> ()  [unwired: 1 in, 9 out]
          }
          frame #1 {
            n259 = local write "PropertyTab"("" ("PropertyTab")) -> ()
          }
        }
      }
      event "ToolbarUpdate": Value Change {
        n260 = event-data() -> ()  [unwired: 7 out]
        n261 = local read "Test"() -> (w338:string)
        n262 = case shown="Default" w338 {
          frame "Test" {
          }
          frame Default {
            n263 = local read "Event Name"() -> (w339:string)
            n264 = case shown="Default" w339 {
              frame "ViewReport" {
              }
              frame Default {
                n265 = control-ref of="This VI"() -> (w341:refnum<vi>)
                n266 = call "CRYUpdate DataView Toolbar.vi"("pVI"=w341) -> ()  [unwired: 11 in]
                n267 = call "CRYPreUpdate Sequence.vi"("EventName"="CurLibUpdate") -> ()  [unwired: 15 in]
              }
            }
          }
        }
      }
    }
    n268 = global read "CRYMain Sub Window Global.vi" "gStop"() -> (w49:bool)
    n269 = Or(x=w49, y="stop") -> (x .or. y?=w45:bool)
  }
  n270 = flat-sequence {
    tunnel: w1 -> [_]
    frame #0 {
      n271 = local write "StateOut"(TRUE ("StateOut")) -> ()
    }
  }
